vi "find_cmd_index.vi"(11 "cmd_name":string) -> (3 "index":u8)   [LabVIEW 2014]
panel:
  in  "files":string[](array[string])=["Wait", "ClawFullOpen", "4BartoGround", "ClawClose", "4BartoCarry", "Turn", "DriveStraight", "4BartoStep", "CollectOn", "CollectOff", "DriveStraight2", "4Barto6", "CollectBlow", "DropStack", "ExitScore", "CloseWheels", "IntakeSense", "StealCan", "Retract", "MaxPower"]
  # "Suck"
  # "Off"
  # "Blow"
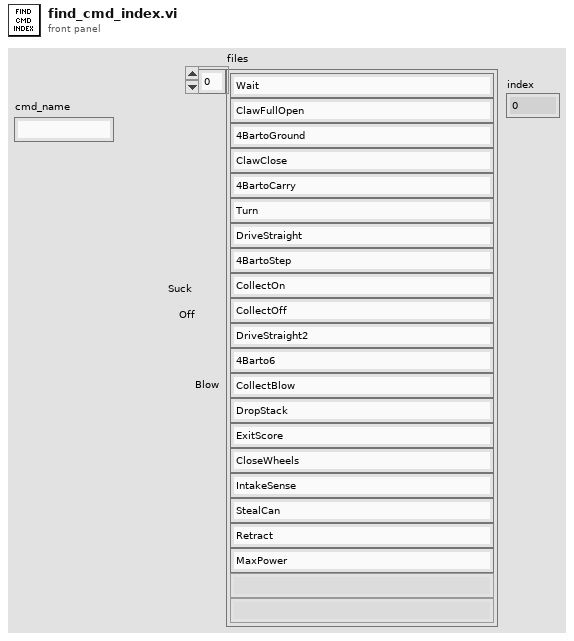
[diagram p1: front panel]
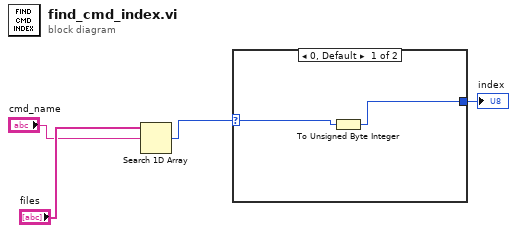
[diagram p0: block diagram]
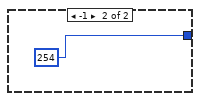
[diagram p2: hidden frame]
diagram:
  n1 = Search 1D Array(1D array="files", element="cmd_name") -> (index of element=w2:i32)  [unwired: 1 in]
  n2 = case shown="0, Default" w2 {
    selector: w2 -> [w6 _]
    tunnel: [w5 u8 254] -> w1
    frame 0, Default {
      n3 = To Unsigned Byte Integer(number=w6) -> (unsigned 8bit integer=w5:u8)
    }
    frame -1 {
    }
  }
  "index" <- w1
